vi "LOG - Copy.vi"(8 "error in (no error)":errorcluster) -> (0 "error out":errorcluster)   [LabVIEW 2014]
uses:
  set_get.ctl
  CMD LOG enum.ctl
  patiant and daq params.ctl
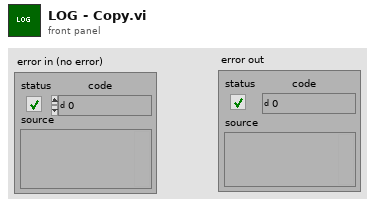
[diagram p1: front panel]
types:
  T1 = typedef "set_get.ctl" = enum16{"Set", "Get"}
  T2 = cluster{"CMD UI":refnum<queue>, "CMD REP":refnum<queue>, "CMD DA":refnum<queue>, "CMD DAQ":refnum<queue>, "CMD LOG":refnum<queue>, "Data LOG":refnum<queue>, "Data Display":refnum<queue>}
  T3 = typedef "patiant and daq params.ctl" = cluster{"DAQ Parameters":cluster{"Sampling rate":dbl, "Max_volt":dbl, "Min_volt":dbl, "DAQmx Physical Channels \nHR,SC":tag, "Resting State":bool}, "Patient Info":cluster{"Patient Name":string, "Patient ID":string, "Patient Age":dbl, "Gender":string}}
  T4 = typedef "CMD LOG enum.ctl" = enum16{"Start Log", "Log", "Stop Log", "Exit"}
  T5 = enum16{"open", "replace", "create", "open or create", "replace or create", "replace or create with confirmation"}
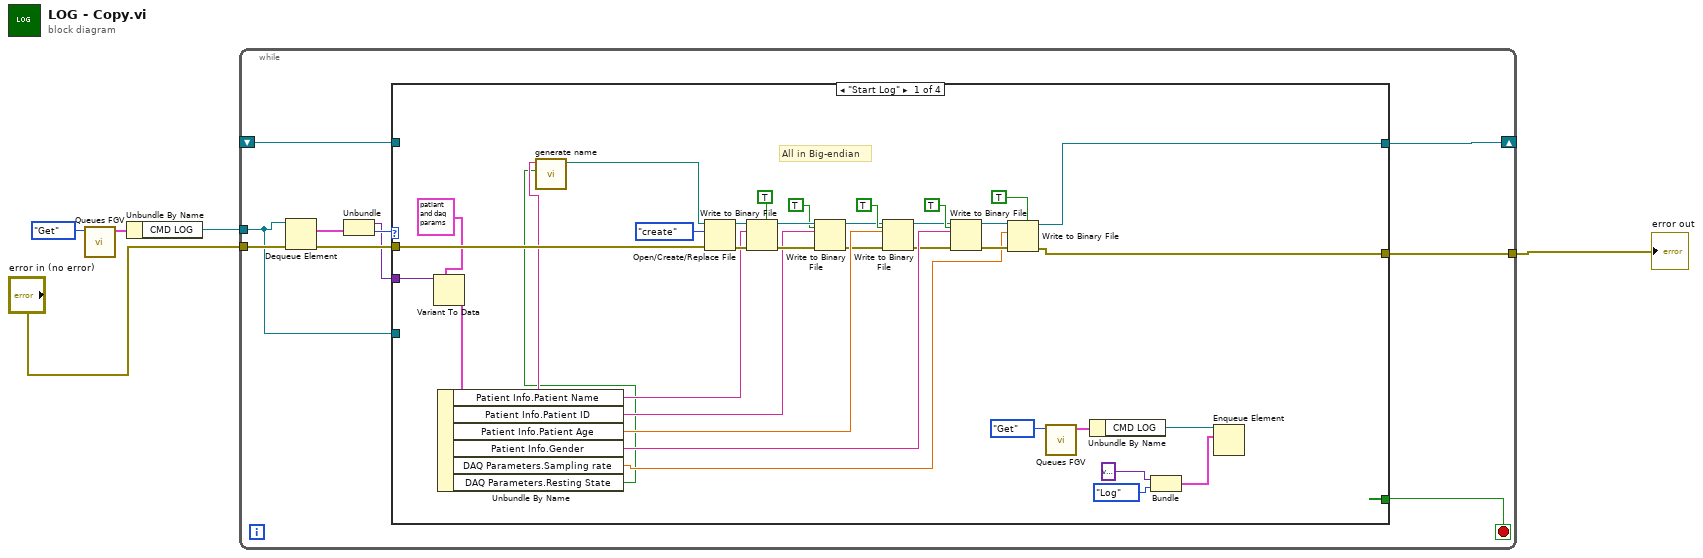
[diagram p0: block diagram]
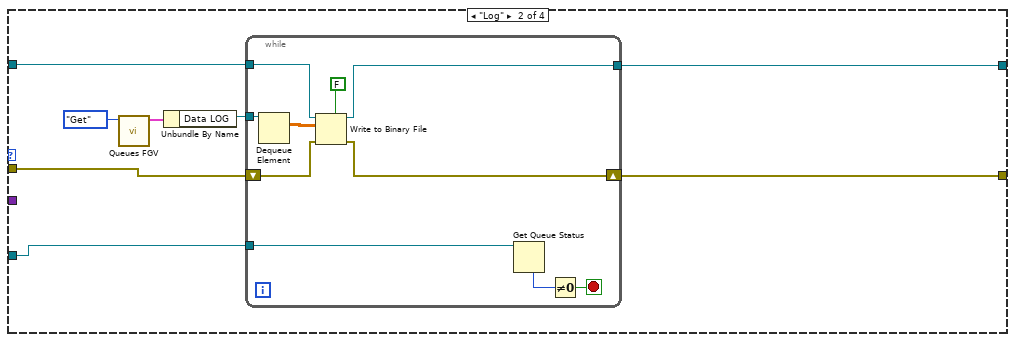
[diagram p2: hidden frame]
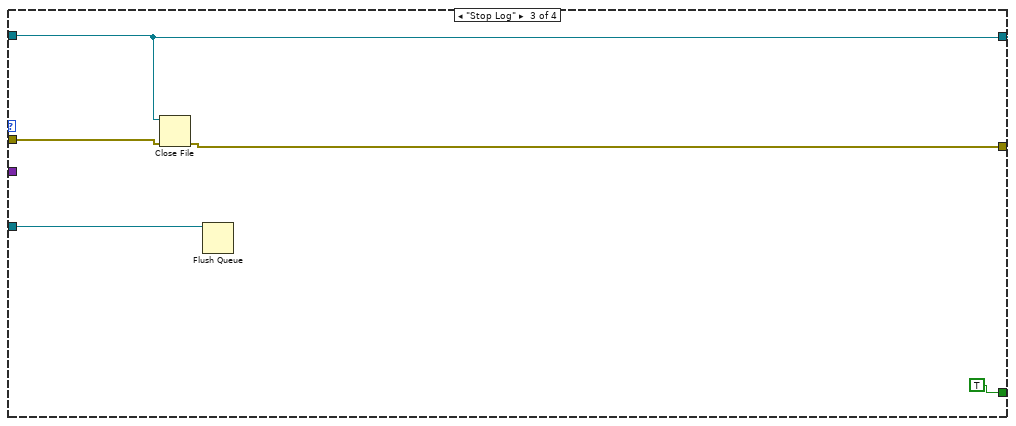
[diagram p3: hidden frame]
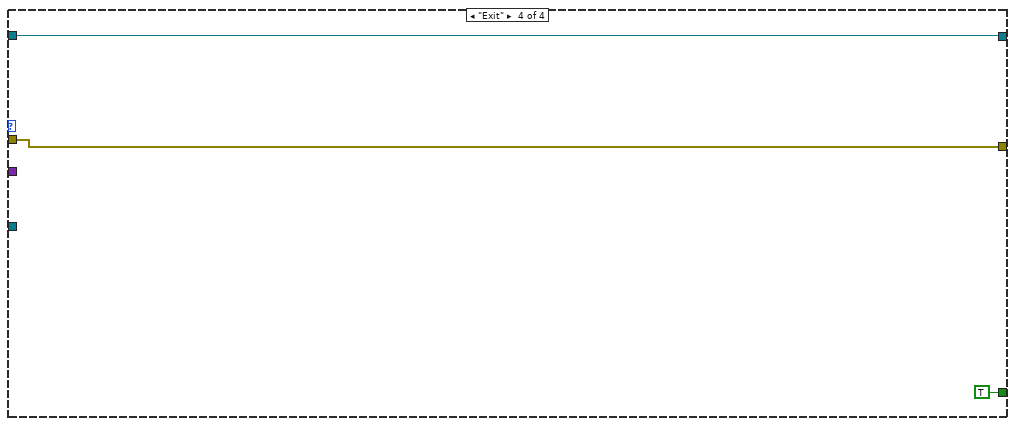
[diagram p4: hidden frame]
diagram:
  n1 = call "Queues FGV.vi"("Enum"=set_get."Get") -> ("Queues"=w4:T2)  [unwired: 10 in]
  n2 = Unbundle By Name(w4) -> ("CMD LOG"=w3:refnum<queue>)
  n3 = while {
    tunnel: w3 -> [w6]
    tunnel: [w12] -> w2
    shift-right: [w11] -> _
    shift-left: _ -> [w10]
    tunnel: "error in (no error)" -> [w8]
    stop <- w9 stop-if-true
    n4 = Dequeue Element(queue=w6, error in (no error)=w8) -> (element=w15:cluster{variant, T4}, error out=w13:errorcluster)  [unwired: 1 in, 2 out]
    n5 = Unbundle(w15) -> (w7:variant, w14:T4)
    n6 = case shown="\"Start Log\"" w14 {
      tunnel: w13 -> [w49 w54 w71 w75]
      tunnel: [w22 w53 w73 w75] -> w12
      tunnel: [w23 w52 w70 w76] -> w11
      tunnel: w10 -> [_ w58 w70 w76]
      tunnel: [_ _ TRUE TRUE] -> w9
      tunnel: w7 -> [w33 _ _ _]
      tunnel: w6 -> [_ w51 w69 _]
      frame "Start Log" {
        # "All in Big-endian"
        n7 = Variant To Data(type=T3 {"DAQ Parameters"={"Sampling rate"=0.0, "Max_volt"=1000.0, "Min_volt"=0.0, "DAQmx Physical Channels \nHR,SC"="", "Resting State"=FALSE}, "Patient Info"={"Patient Name"="", "Patient ID"="", "Patient Age"=0.0, "Gender"=""}} ("The Cluster"), Variant=w33) -> (data=w32:T3)  [unwired: 1 in, 1 out]
        n8 = Unbundle By Name(w32) -> ("Patient Info.Patient Name"=w18:string, "Patient Info.Patient ID"=w43:string, "Patient Info.Patient Age"=w40:dbl, "Patient Info.Gender"=w36:string, "DAQ Parameters.Sampling rate"=w21:dbl, "DAQ Parameters.Resting State"=w16:bool)
        n9 = call "generate name.vi"("rest (T) active (F)"=w16, "Patient Name"=w18) -> ("appended path"=w19:path)  [unwired: 9 in]
        n10 = Open/Create/Replace File(file path (use dialog)=w19, error in=w49, operation (0:open)=T5."create") -> (refnum out=w48:refnum<file>, error out=w47:errorcluster)  [unwired: 3 in, 1 out]
        n11 = Write to Binary File(file (use dialog)=w48, data=w18, error in=w47, 5:TRUE ("prepend array or string size? (T)")) -> (refnum out=w44:refnum<file>, error out=w45:errorcluster)  [unwired: 2 in, 1 out]
        n12 = Write to Binary File(file (use dialog)=w44, data=w43, error in=w45, 5:TRUE ("prepend array or string size? (T)")) -> (refnum out=w38:refnum<file>, error out=w39:errorcluster)  [unwired: 2 in, 1 out]
        n13 = Write to Binary File(file (use dialog)=w38, data=w40, error in=w39, 5:TRUE ("prepend array or string size? (T)")) -> (refnum out=w35:refnum<file>, error out=w34:errorcluster)  [unwired: 2 in, 1 out]
        n14 = Write to Binary File(file (use dialog)=w35, data=w36, error in=w34, 5:TRUE ("prepend array or string size? (T)")) -> (refnum out=w24:refnum<file>, error out=w25:errorcluster)  [unwired: 2 in, 1 out]
        n15 = Write to Binary File(file (use dialog)=w24, data=w21, error in=w25, 5:TRUE ("prepend array or string size? (T)")) -> (refnum out=w23:refnum<file>, error out=w22:errorcluster)  [unwired: 2 in, 1 out]
        n16 = call "Queues FGV.vi"("Enum"=set_get."Get") -> ("Queues"=w31:T2)  [unwired: 10 in]
        n17 = Unbundle By Name(w31) -> ("CMD LOG"=w29:refnum<queue>)
        n18 = Bundle(variant, "Enum"=CMD_LOG_enum."Log") -> (w26:cluster{variant, "Enum":T4})  [unwired: 1 in]
        n19 = Enqueue Element(queue=w29, element=w26) -> ()  [unwired: 2 in, 3 out]
      }
      frame "Log" {
        n20 = call "Queues FGV.vi"("Enum"=set_get."Get") -> ("Queues"=w57:T2)  [unwired: 10 in]
        n21 = Unbundle By Name(w57) -> ("Data LOG"=w55:refnum<queue>)
        n22 = while {
          tunnel: w58 -> [w68]
          tunnel: w55 -> [w67]
          tunnel: [w63] -> w52
          shift-right: [w64] -> w53
          shift-left: w54 -> [w65]
          tunnel: w51 -> [w60]
          stop <- w61 stop-if-true
          n23 = Dequeue Element(queue=w67) -> (element=w66:dbl[][])  [unwired: 2 in, 3 out]
          n24 = Write to Binary File(file (use dialog)=w68, data=w66, error in=w65, 5:FALSE ("prepend array or string size? (T)")) -> (refnum out=w63:refnum<file>, error out=w64:errorcluster)  [unwired: 2 in, 1 out]
          n25 = Get Queue Status(queue=w60) -> (# elements in queue=w62:i32)  [unwired: 2 in, 7 out]
          n26 = Not Equal To 0?(x=w62) -> (x != 0?=w61:bool)
        }
      }
      frame "Stop Log" {
        n27 = Close File(refnum=w70, error in=w71) -> (error out=w73:errorcluster)  [unwired: 1 out]
        n28 = Flush Queue(queue=w69) -> ()  [unwired: 1 in, 3 out]
      }
      frame "Exit" {
      }
    }
  }
  "error out" <- w2
